vi "DialogDefineChannel.vi"(8 "error in":errorcluster, 9 "Input String":string, 10 "Available Paths":string[](array[string]), 11 "Available Refs":T1[](array[typedef]) format="%.0x") -> (0 "error out":errorcluster, 1 "Selected Path":string, 2 "Selected Ref":T1 format="%.0x", 3 "Cancelled?":bool)   [LabVIEW 2024, in "Embedded TDMS Logger System Explorer.lvlib"]
doc: "Requests the user to specify a specific channel as the channel given by the string path was not found."
uses:
  Embedded TDMS Logger System Explorer.lvlib
  <vilib>/NI VeriStand/Custom Device API/Custom Device Item Ref.ctl
  <vilib>/NI VeriStand/Custom Device API/Custom Device API.lvlib
panel:
  in  "Channel":string(combo)
  in  "OK Button":bool
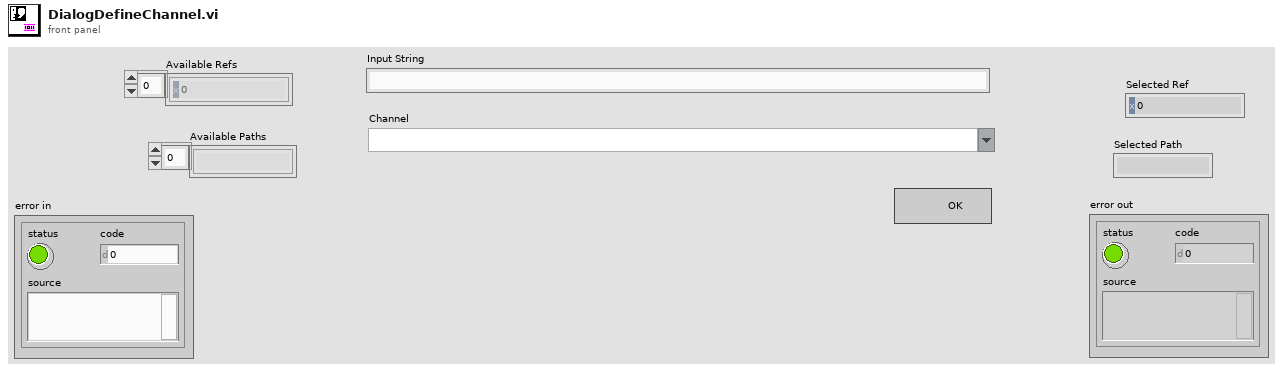
[diagram p1: front panel]
types:
  T1 = typedef "Custom Device API.lvlib/Custom Device Item Ref.ctl" = u64
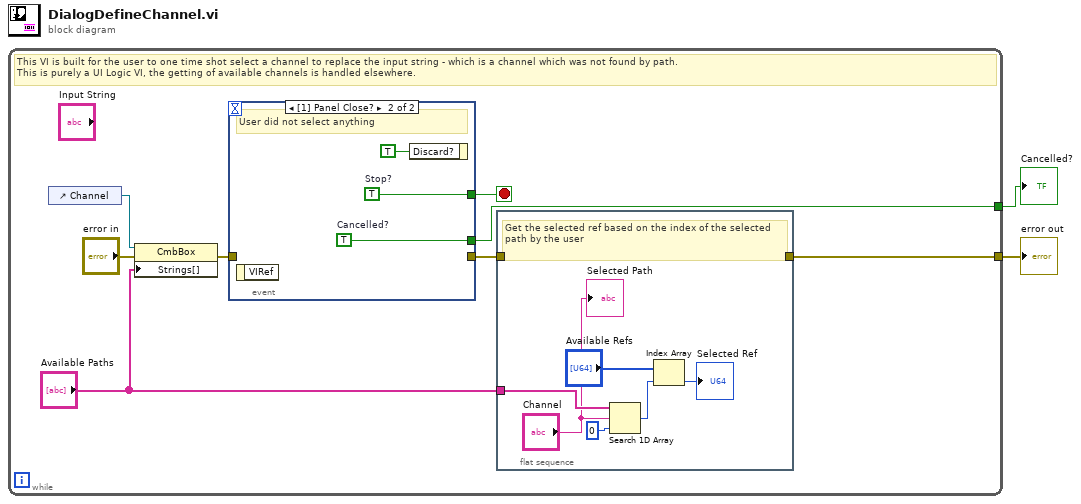
[diagram p0: block diagram]
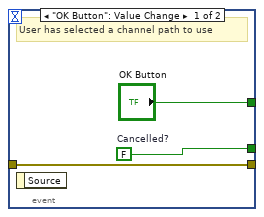
[diagram p2: hidden frame]
diagram:
  n1 = while {
    tunnel: [w9] -> w2
    tunnel: [w8] -> w1
    stop <- w10 stop-if-true
    # "This VI is built for the user to one time shot select a channel to replace the input string - which is a channel which was not found by path.\nThis is purely a UI Logic VI, the getting of available channels is handled elsewhere."
    n2 = control-ref of="Channel"() -> (w4:refnum<vi>)
    n3 = property class="CmbBox"(reference=w4, error in="error in", "Strings[]"="Available Paths") -> (error out=w5:errorcluster)  [unwired: 1 out]
    n4 = event shown="[1] Panel Close?" {
      selector: _ -> [_ _]
      dyn-events: _ -> [_ _]
      timeout: _ -> [_ _]
      tunnel: ["OK Button" w22] -> w10
      tunnel: [w20 w21] -> w9
      tunnel: [w18 _] -> w6
      tunnel: w5 -> [w18 _]
      event "OK Button": Value Change {
        w20 = FALSE  # Cancelled?
        # "User has selected a channel path to use"
        n5 = event-data() -> ()  [unwired: 1 in, 1 out]
      }
      event Panel Close? {
        w21 = TRUE  # Cancelled?
        w22 = TRUE  # Stop?
        # "User did not select anything"
        n6 = event-data() -> ()  [unwired: 1 in, 1 out]
        n7 = event-data("Discard?"=TRUE) -> ()  [unwired: 1 in, 1 out]
      }
    }
    n8 = flat-sequence {
      tunnel: w6 -> [w17]
      tunnel: [w17] -> w8
      tunnel: "Available Paths" -> [w14]
      frame #0 {
        # "Get the selected ref based on the index of the selected path by the user"
        n9 = Search 1D Array(1D array=w14, element="Channel", start index (0)=0) -> (index of element=w15:i32)
        n10 = Index Array(array="Available Refs", index=w15) -> (element=→"Selected Ref":T1)
        "Selected Path" <- "Channel"
      }
    }
  }
  "Cancelled?" <- w2
  "error out" <- w1
